vi "write frame to acquisition file - subvi.vi"(1 "Pixel depth":u32(ring) items=["8 bits", "16 bits", "Float", "Complex", "RGB", "HSL"], 4 "Frames per acquisition file":u32, 7 "Offset table in":cluster{"offset":i32, "file number":u8}[](array[cluster]), 8 "Error In":errorcluster, 9 "Image In":T1, 10 "Sequence files handle":T2, 11 "Last frame number written in":u32) -> (0 "Error Out":errorcluster, 2 "Last frame number written out":u32, 3 "Stop":bool, 5 "Offset table out":cluster{"offset":i32, "file number":u8}[](array[cluster]))   [LabVIEW 2014]
doc: "Writes binary data of an image to the acquisition files which are found in RAID Root Path. Only image pixel values of U8 and I16 are written. I16 is the default."
uses:
  <vilib>/vision/Image Controls.llb/IMAQ Image.ctl
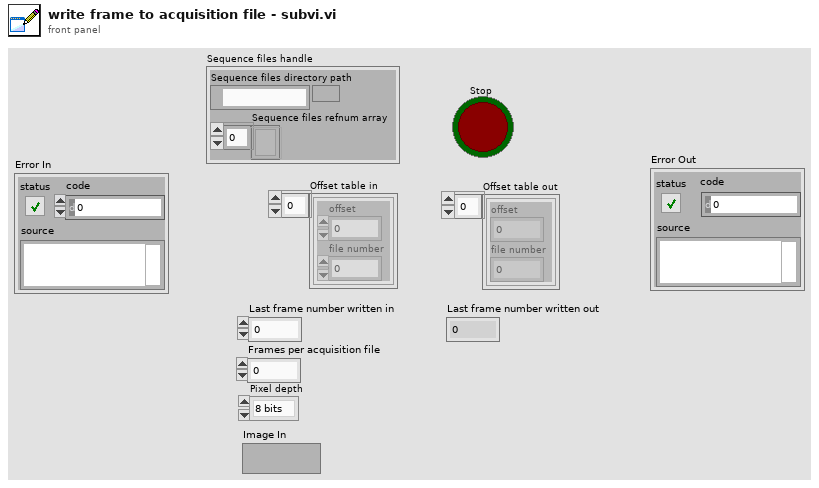
[diagram p1: front panel]
types:
  T1 = typedef "IMAQ Image.ctl" = refnum<image>
  T2 = cluster{"Sequence files directory path":path, "Sequence files refnum array":refnum<file>[]}
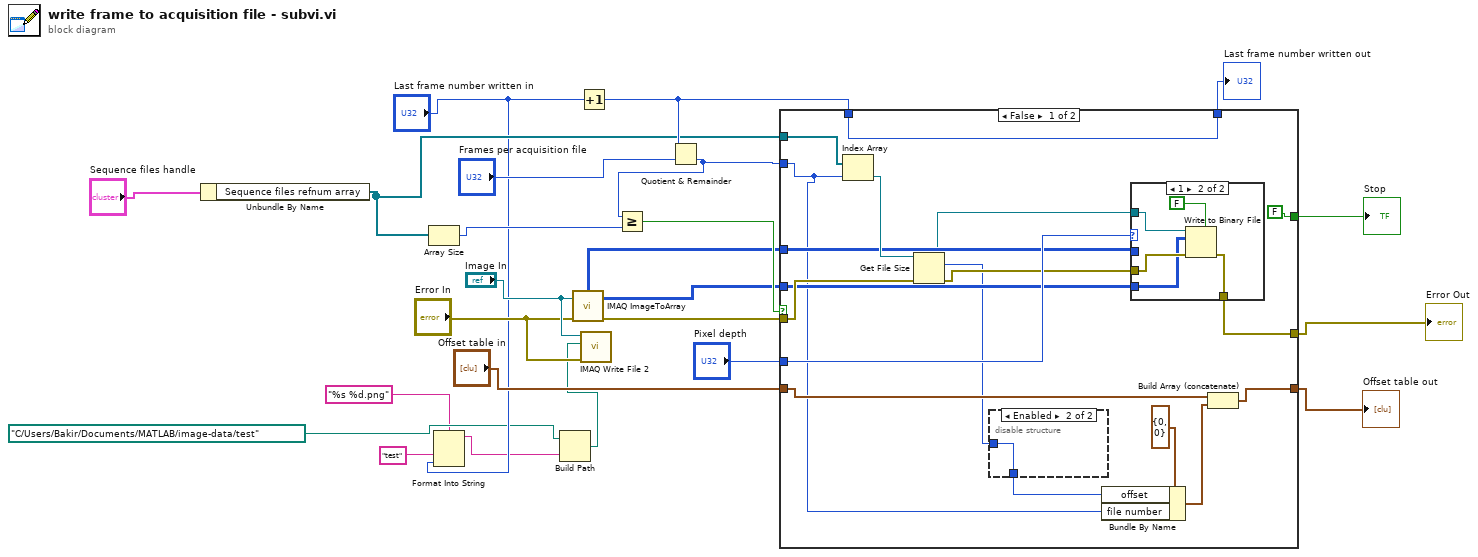
[diagram p0: block diagram]
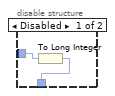
[diagram p2: hidden frame]
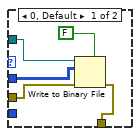
[diagram p3: hidden frame]
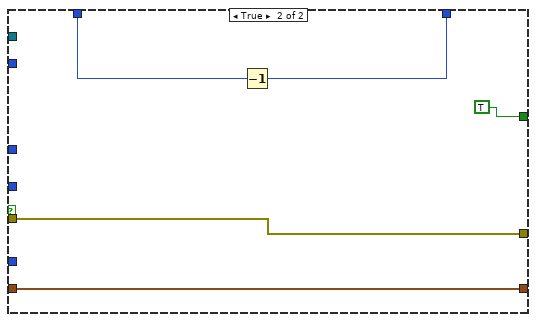
[diagram p4: hidden frame]
diagram:
  n1 = Unbundle By Name("Sequence files handle") -> ("Sequence files refnum array"=w9:refnum<file>[])
  n2 = Array Size(array=w9) -> (size(s)=w23:i32)
  n3 = Format Into String(format string="%s %d.png", "test", "Last frame number written in") -> (resulting string=w5:string)  [unwired: 2 in, 1 out]
  n4 = Build Path(base path=path "C:/Users/Bakir/Documents/MATLAB/image-data/test" ("File Path"), name or relative path=w5) -> (appended path=w3:path)
  n5 = call "IMAQ ImageToArray"("error in (no error)"="Error In", "Image"="Image In") -> ("error out"=w14:errorcluster, "Image Pixels (U8)"=w15:u8[][], "Image Pixels (I16)"=w16:i16[][])  [unwired: 2 in, 2 out]
  n6 = Increment(x="Last frame number written in") -> (x+1=w17:u32)
  n7 = call-poly "IMAQ Write File 2"("error in (no error)"="Error In", "File Path"=w3, "Image"="Image In") -> ()  [unwired: 7 in, 2 out]
  n8 = Quotient & Remainder(x=w17, y="Frames per acquisition file") -> (floor(x/y)=w18:u32)  [unwired: 1 out]
  n9 = Greater Or Equal?(x=w18, y=w23) -> (x >= y?=w21:bool)
  n10 = case shown="False" w21 {
    tunnel: "Offset table in" -> [w33 w60]
    tunnel: "Pixel depth" -> [w38 _]
    tunnel: w18 -> [w30 _]
    tunnel: w17 -> [w41 w58]
    tunnel: w16 -> [w35 _]
    tunnel: w15 -> [w36 _]
    tunnel: w14 -> [w40 w59]
    tunnel: [w27 w60] -> w13
    tunnel: [w26 w59] -> w11
    tunnel: [w41 w57] -> w12
    tunnel: [FALSE TRUE] -> w10
    tunnel: w9 -> [w42 _]
    frame False {
      n11 = Index Array(array=w42, index=w30) -> (element=w39:refnum<file>)
      n12 = Get File Size(file=w39, error in=w40) -> (refnum out=w34:refnum<file>, size (in bytes)=w32:i64, 0:w37:errorcluster)
      n13 = disable-structure shown="Enabled" {
        disable-tunnel: w32 -> [w44 w45]
        disable-tunnel: [w43 w45] -> w29
        frame Disabled {
          n14 = To Long Integer(number=w44) -> (32bit integer=w43:i32)
        }
        frame Enabled {
        }
      }
      n15 = Bundle By Name(cluster=cluster{"offset":i32, "file number":u8} {"offset"=0, "file number"=0} ("Cluster"), "offset"=w29, "file number"=w30) -> (w28:cluster{"offset":i32, "file number":u8})
      n16 = case shown="1" w38 {
        tunnel: w37 -> [w49 w54]
        tunnel: w36 -> [w47 _]
        tunnel: w35 -> [_ w52]
        tunnel: w34 -> [w50 w55]
        tunnel: [w48 w53] -> w26
        frame 0, Default {
          n17 = Write to Binary File(file (use dialog)=w50, data=w47, error in=w49, 5:FALSE ("prepend array or string size? (T)")) -> (error out=w48:errorcluster)  [unwired: 1 in, 3 out]
        }
        frame 1 {
          n18 = Write to Binary File(file (use dialog)=w55, data=w52, error in=w54, 5:FALSE ("prepend array or string size? (T)")) -> (error out=w53:errorcluster)  [unwired: 4 out]
        }
      }
      n19 = Build Array (concatenate)(w33, w28) -> (w27:cluster{"offset":i32, "file number":u8}[])
    }
    frame True {
      n20 = Decrement(x=w58) -> (x-1=w57:u32)
    }
  }
  "Offset table out" <- w13
  "Last frame number written out" <- w12
  "Error Out" <- w11
  "Stop" <- w10
